vi "ReadFIFO.vi"(6 "dt of Timeloop(ms)":i64=5, 7 "Stop":bool, 8 "Count":dbl, 9 "Buffer factor":dbl=1.5, 10 "FIFO size":u32=3000, 11 "RT FIFO":refnum<k33>) -> (0 "Stop write file":bool, 1 "element out":dbl[](array[numeric])=[-1800.0, 0.0, -1800.0, 0.0, -1800.0, 0.0, -1800.0, 0.0, -1800.0, 0.0, -1800.0, 0.0, -1800.0, 0.0, -1800.0, 0.0, 1.0, 1.0, 1.0, 1.0, 0.0, 0.0, 0.0, 0.0, 0.0, 0.0, 28.52127742767334, -0.059714317321777344, 0.08044290542602539, 1.058915615081787, 0.9604449272155762, 0.9433765411376953, 0.9154763221740723, 0.9282774925231934, 0.9433765411376953, 0.9295907020568848], 2 "# elements":u32=513, 3 "RT FIFO (to delete)":refnum<k33>, 4 "Stop read file":bool)   [LabVIEW 2019]
panel:
  out "empty?":bool
  out "Read Count":i32=961
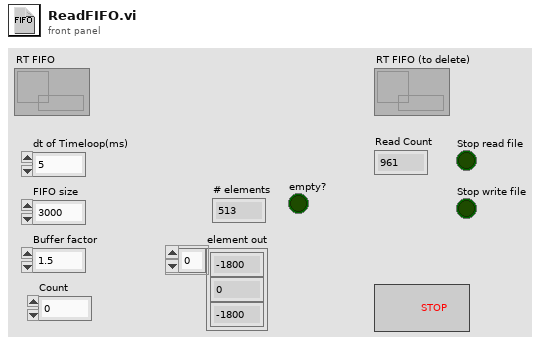
[diagram p1: front panel]
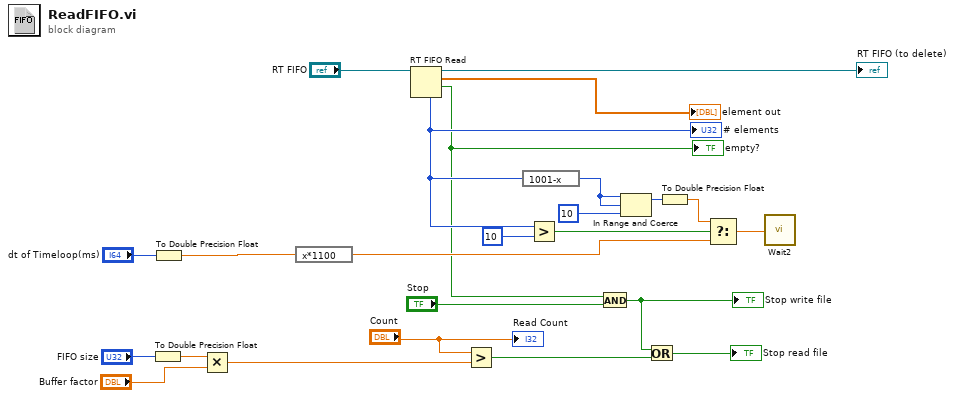
[diagram p0: block diagram]
diagram:
  n1 = To Double Precision Float(number="FIFO size") -> (double precision float=w18:dbl)
  n2 = To Double Precision Float(number="dt of Timeloop(ms)") -> (double precision float=w17:dbl)
  n3 = Multiply(x=w18, y="Buffer factor") -> (x*y=w20:dbl)
  n4 = expression code="x*1100"(w17) -> (w22:dbl)
  n5 = RT FIFO Read(0:"RT FIFO") -> (7:w9:u32, 8:→"RT FIFO (to delete)":refnum<k33>, 9:→"element out":dbl[], 10:w4:bool)  [unwired: 3 in, 1 out]
  "# elements" <- w9
  "empty?" <- w4
  n6 = Greater?(x="Count", y=w20) -> (0:w11:bool)
  n7 = expression code="1001-x"(w9) -> (w7:u32)
  n8 = Greater?(x=w9, y=u32 10) -> (0:w6:bool)
  n9 = And(x=w4, y="Stop") -> (x .and. y?=w14:bool)
  "Stop write file" <- w14
  n10 = In Range and Coerce(upper limit=w7, x=w7, lower limit=u32 10) -> (coerced(x)=w3:u32)  [unwired: 1 out]
  n11 = Or(x=w14, y=w11) -> (x .or. y?=→"Stop read file":bool)
  n12 = To Double Precision Float(number=w3) -> (double precision float=w2:dbl)
  n13 = Select(t=w2, s=w6, f=w22) -> (s? t:f=w12:dbl)
  n14 = call "Wait2"("Count(uSec)"=w12) -> ()  [unwired: 1 out]
  "Read Count" <- "Count"
